vi "Set PGI Attribute.vi"(7 "para3":cluster{} caption="空簇", 8 "error in (no error)":errorcluster caption="错误输入（无错误）", 9 "attribute":i32, 10 "pgiDevNum":i32, 11 "pgiType":i32) -> (0 "error out":errorcluster caption="错误输出", 3 "function return":i32)   [LabVIEW 2018]
doc: "extern int APSxSetPGIAttribute (int pgiType, int pgiDevNum, IN int attribute, IN ...);"
uses:
  APSx.dll/APSx.dll
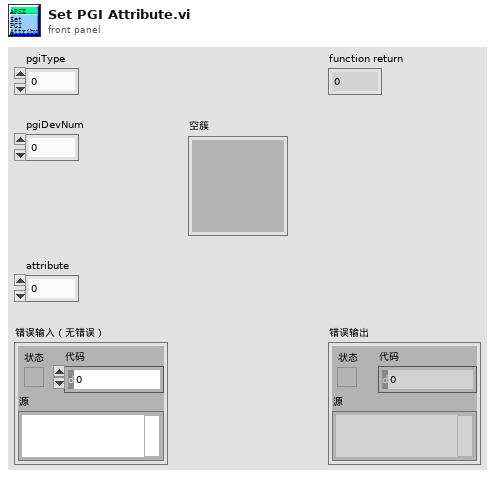
[diagram p1: front panel]
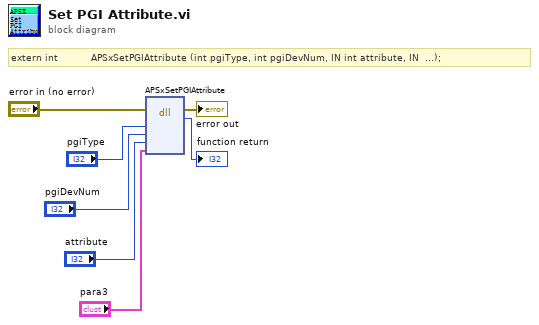
[diagram p0: block diagram]
diagram:
  # "extern int           APSxSetPGIAttribute (int pgiType, int pgiDevNum, IN int attribute, IN  ...);"
  n1 = dll-call lib="PTH2[abs D项目Feng恒隆项目Labview传感器对中台SourcesAPSx.dllAPSx.*" fn="APSxSetPGIAttribute"(error in="error in (no error)", "pgiType"="pgiType", "pgiDevNum"="pgiDevNum", "attribute"="attribute", "para3"="para3") -> (error out=→"error out":errorcluster, →"function return":i32)  [unwired: 6 in, 1 out]
